vi "Second Test.vi"() -> ()   [LabVIEW 2017]
uses:
  Assertion/Assertion.lvlib
panel:
  out "error out":errorcluster
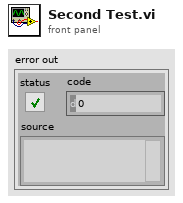
[diagram p1: front panel]
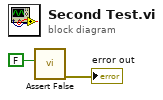
[diagram p0: block diagram]
diagram:
  n1 = call "Assert False.vi"("Condition"=FALSE) -> ("error out"=→"error out":errorcluster)  [unwired: 10 in]
